vi "Archive files move dir.vi"(5 "hours old date mod(hours)":u8=255, 6 "error in":errorcluster, 7 "File path input cluster":T1={"Archive Location"=path "", "Archive Location 2"=path "<Not A Path>", "OutPut Path"=path "", "Directory(s) To Scan Files"=[]}, 8 "File Management":T2, 9 "Timing True to archive":bool) -> (0 "ErrorArray":errorcluster[][](array[cluster]), 1 "File path input cluster (out)":T1={"Archive Location"=path "", "Archive Location 2"=path "<Not A Path>", "OutPut Path"=path "", "Directory(s) To Scan Files"=[]})   [LabVIEW 2012]
uses:
  Controls/File Management.ctl
  Controls/File Path directories.ctl
  <vilib>/Utility/sysdir.llb/System Directory Type.ctl
panel:
  # "File Handling Method"
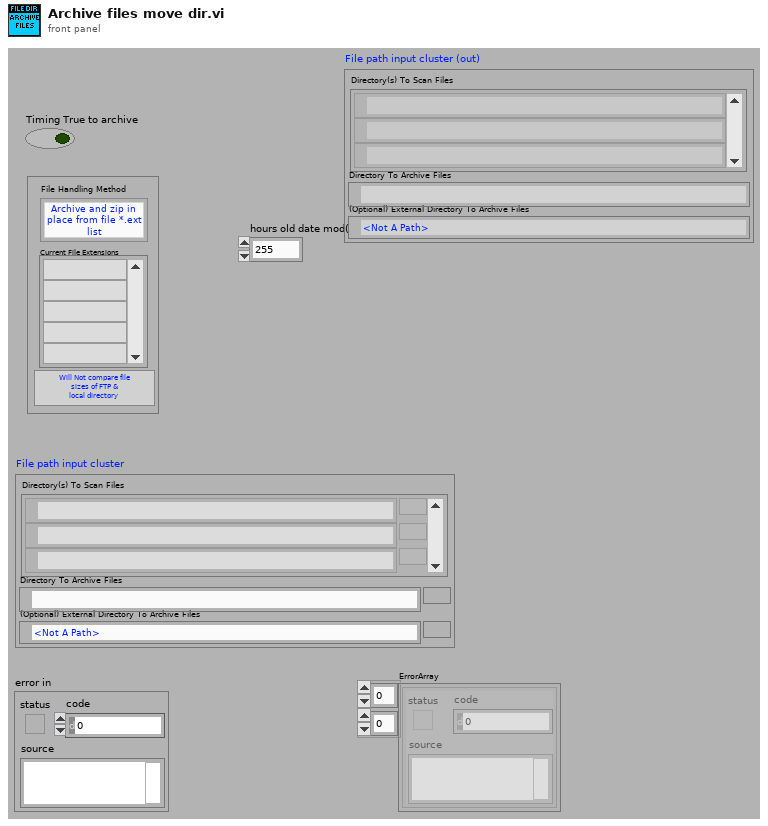
[diagram p1: front panel]
types:
  T1 = typedef "File Path directories.ctl" = cluster{"Archive Location":path, "Archive Location 2":path, "OutPut Path":path, "Directory(s) To Scan Files":path[]}
  T2 = typedef "File Management.ctl" = cluster{"Comp File Size":bool, "File Handle Method":enum16{"Archive and zip in place from file *.ext list", "Archive and zip ALL file Types to archive directory", "Archive and zip to archive directory from file *.ext list", "Perform no file management"}, "file extention list":string[]}
  T3 = enum16{"Archive and zip in place from file *.ext list", "Archive and zip ALL file Types to archive directory", "Archive and zip to archive directory from file *.ext list", "Perform no file management"}
  T4 = typedef "System Directory Type.ctl" = i32
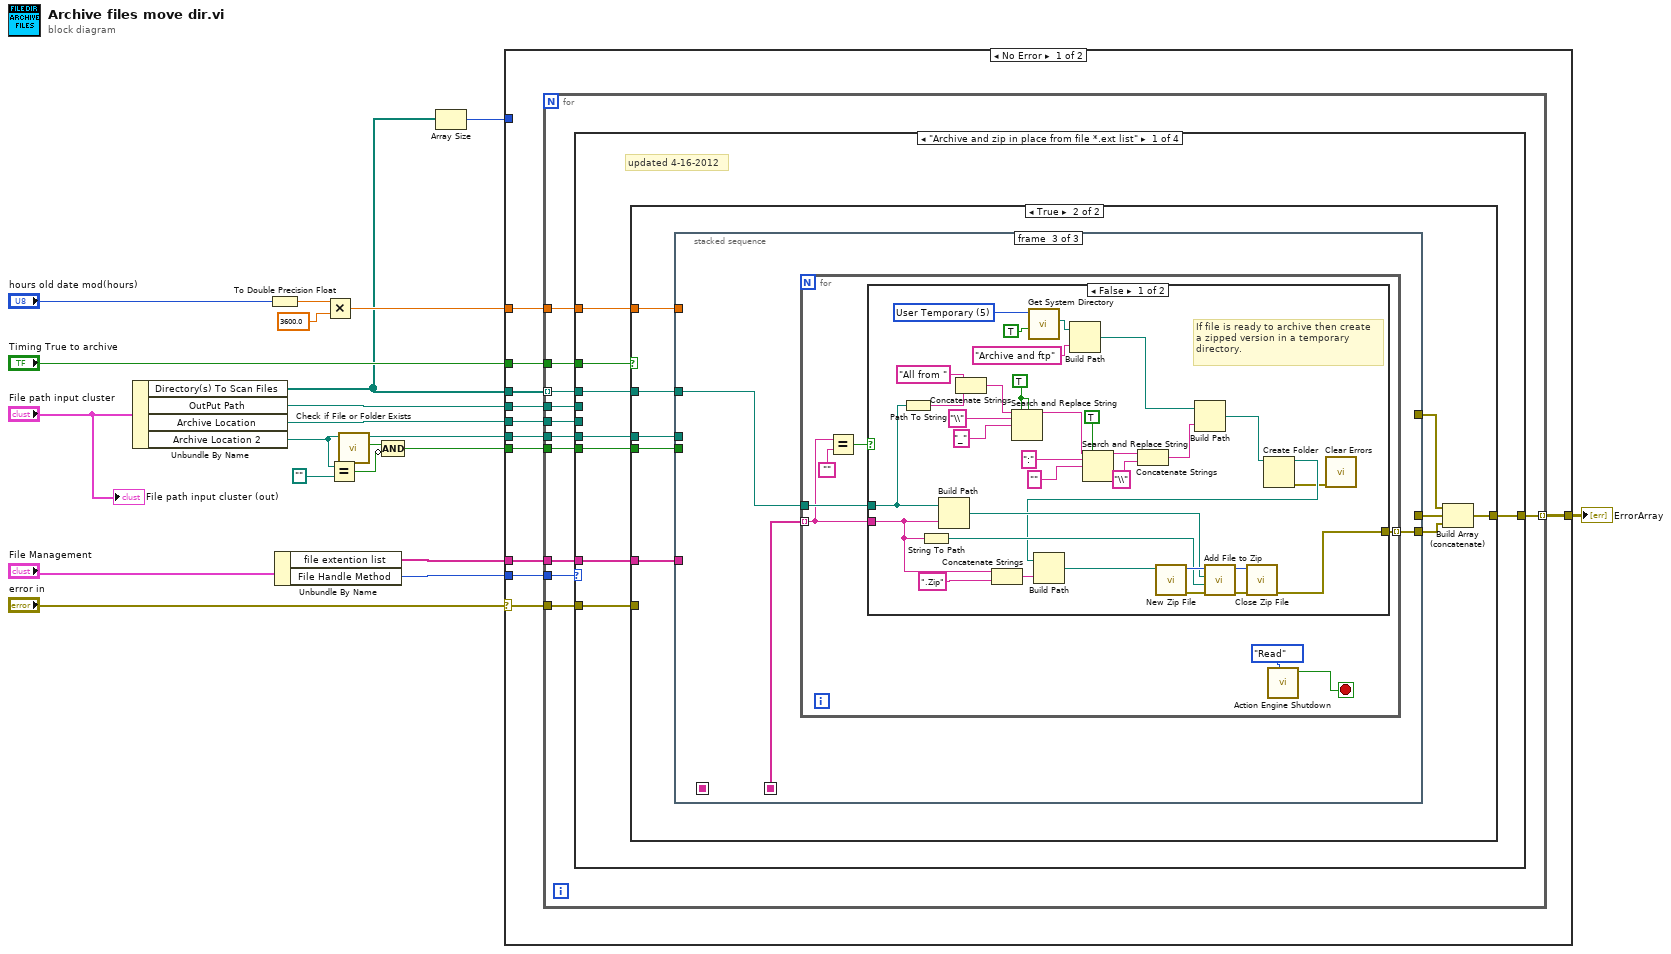
[diagram p0: block diagram]
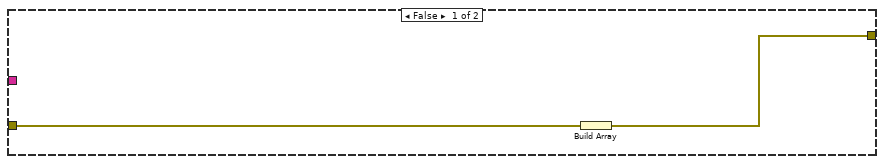
[diagram p2: hidden frame]
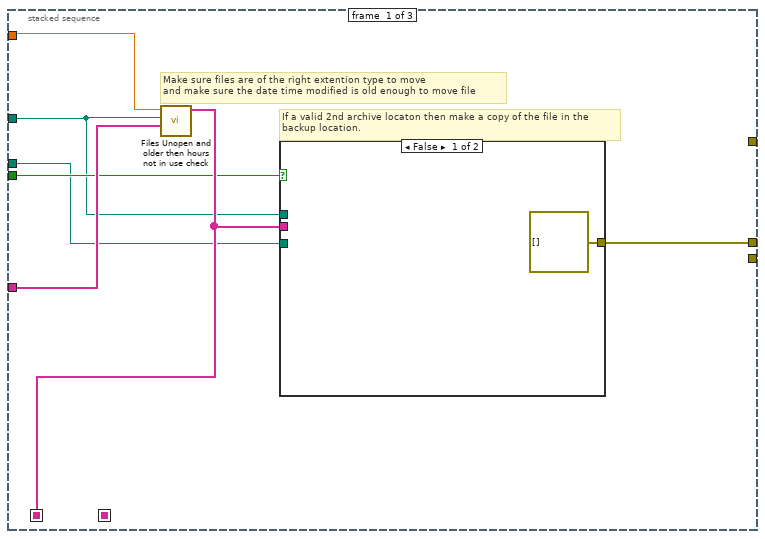
[diagram p3: hidden frame]
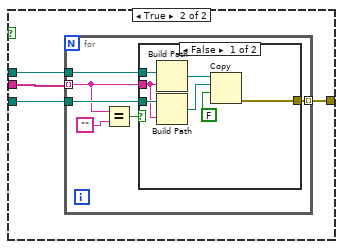
[diagram p4: hidden frame]
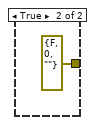
[diagram p5: hidden frame]
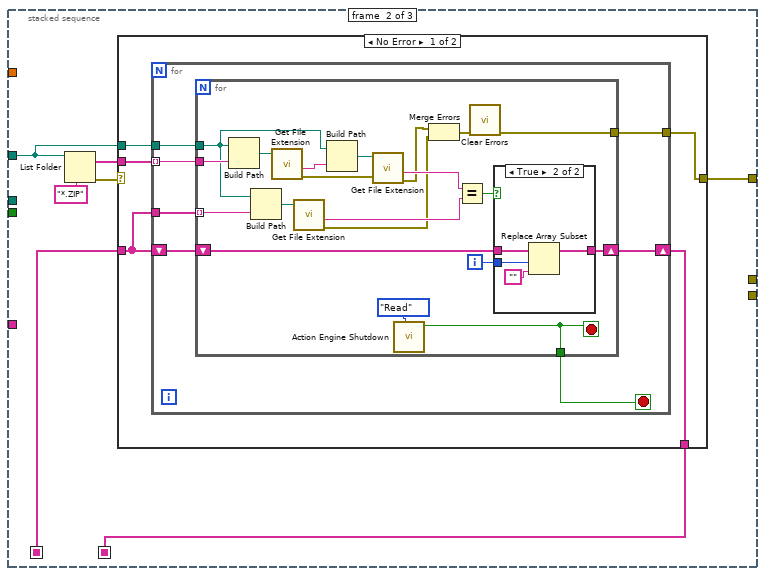
[diagram p6: hidden frame]
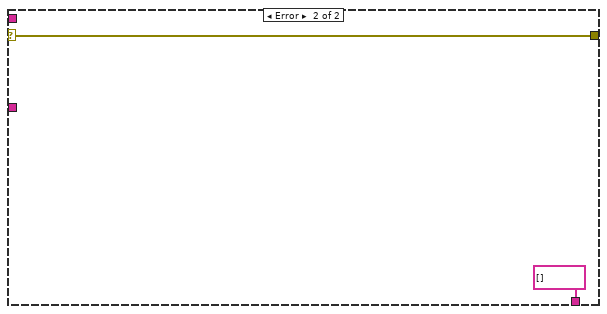
[diagram p8: hidden frame]
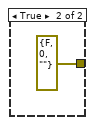
[diagram p9: hidden frame]
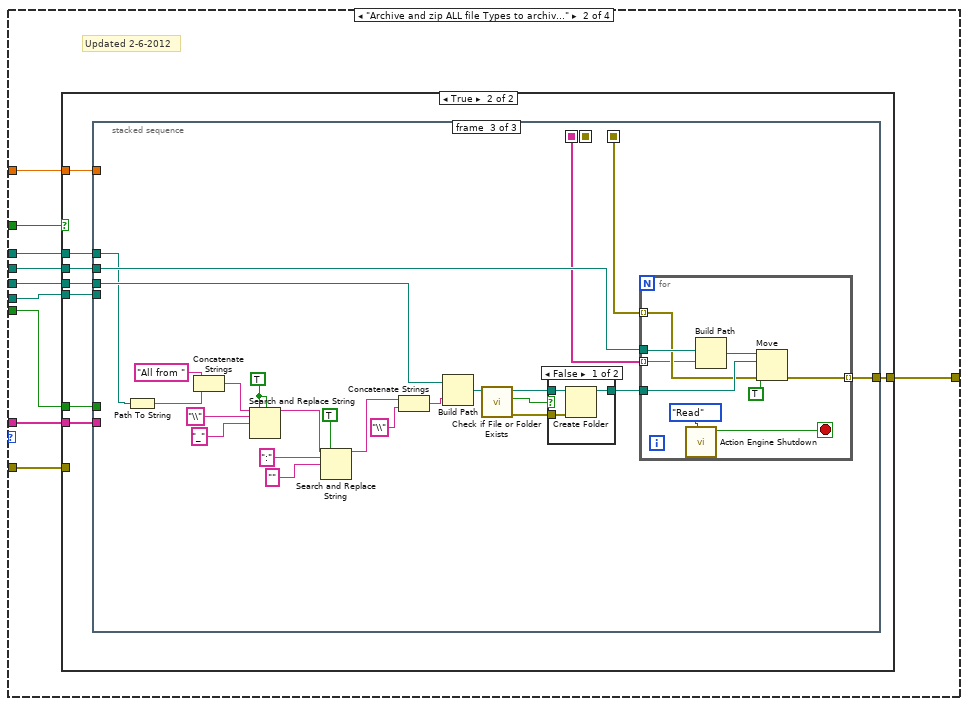
[diagram p10: hidden frame]
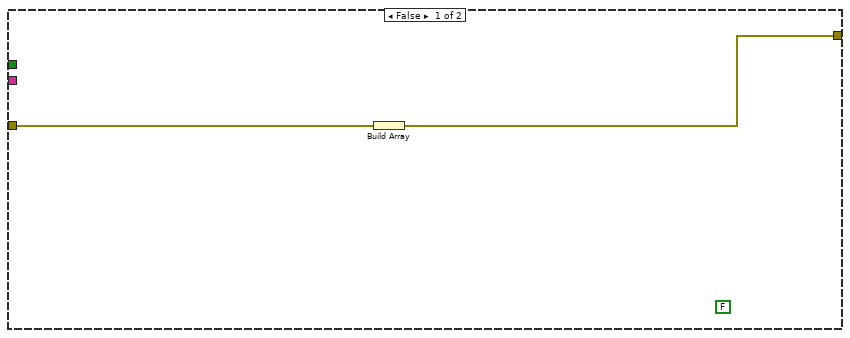
[diagram p11: hidden frame]
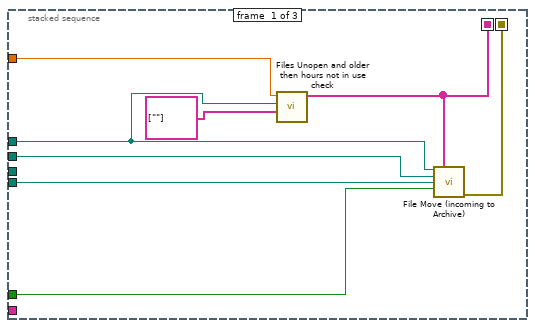
[diagram p12: hidden frame]
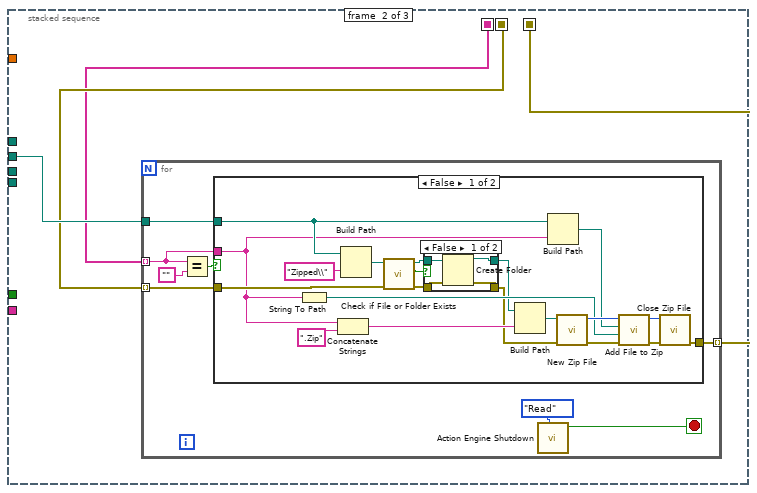
[diagram p13: hidden frame]
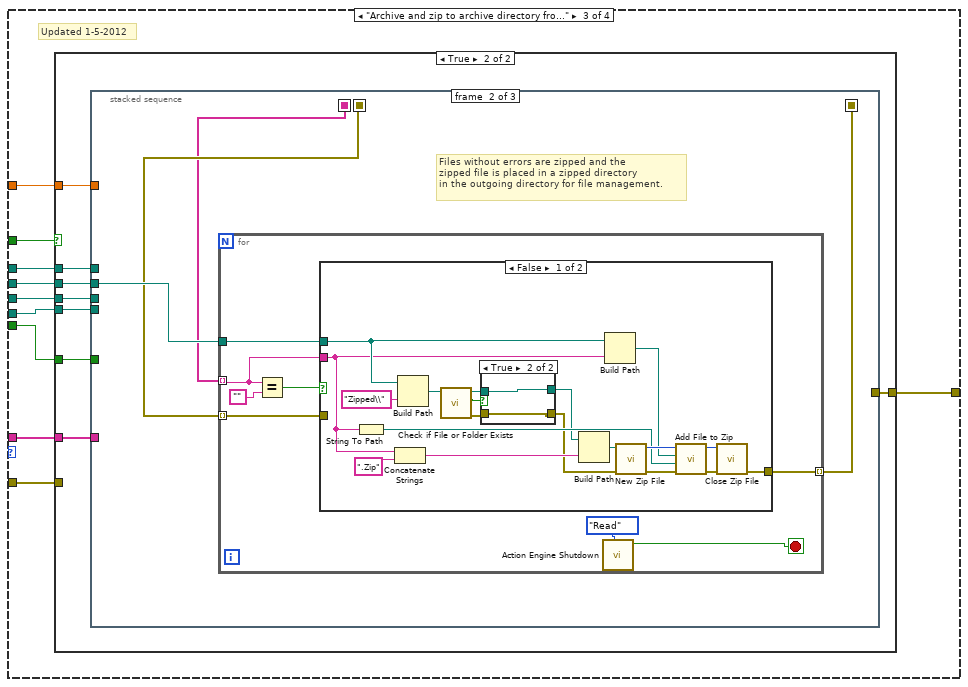
[diagram p17: hidden frame]
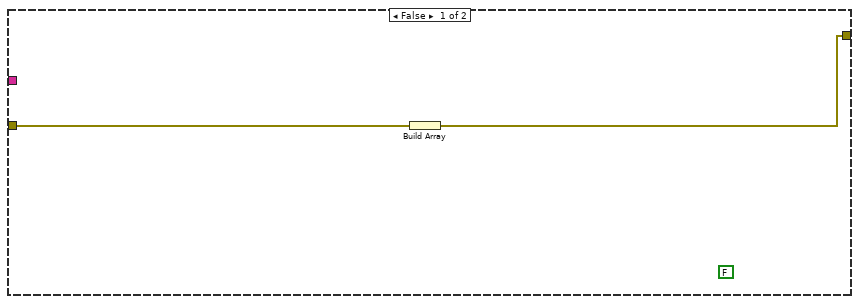
[diagram p18: hidden frame]
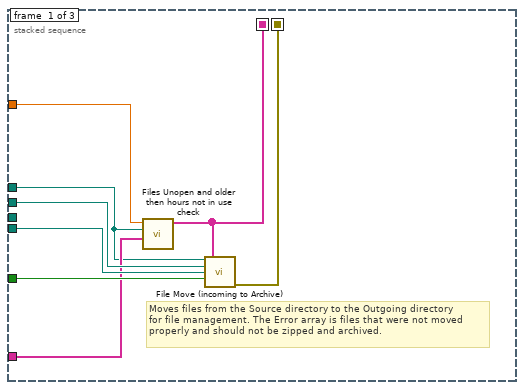
[diagram p19: hidden frame]
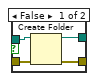
[diagram p20: hidden frame]
diagram:
  n1 = Unbundle By Name("File path input cluster") -> ("Directory(s) To Scan Files"=w3:path[], "OutPut Path"=w12:path, "Archive Location"=w11:path, "Archive Location 2"=w17:path)
  n2 = To Double Precision Float(number="hours old date mod(hours)") -> (double precision float=w6:dbl)
  n3 = Unbundle By Name("File Management") -> ("file extention list"=w18:string[], "File Handle Method"=w20:T3)
  n4 = Multiply(x=w6, y=3600.0) -> (x*y=w7:dbl)
  n5 = Equal?(x=w17, y=path "") -> (x = y?=w14:bool)
  n6 = call <vilib>:"Check if File or Folder Exists.vi"("path"=w17) -> ("file or folder exists?"=w15:bool, "dup path"=w10:path)  [unwired: 8 in, 1 out]
  n7 = Compound Arithmetic op=AND(w15, invert w14) -> (w9:bool)
  n8 = Array Size(array=w3) -> (size(s)=w2:i32)
  n9 = case shown="No Error" "error in" {
    selector: "error in" -> [w22 w381]
    tunnel: "Timing True to archive" -> [w32 _]
    tunnel: [w23 w379] -> w1
    tunnel: w20 -> [w31 _]
    tunnel: w18 -> [w30 _]
    tunnel: w3 -> [w29 _]
    tunnel: w12 -> [w28 _]
    tunnel: w11 -> [w27 _]
    tunnel: w10 -> [w26 _]
    tunnel: w9 -> [w25 _]
    tunnel: w7 -> [w24 _]
    tunnel: w2 -> [_ _]
    frame No Error {
      n10 = for {
        tunnel: w32 -> [w43]
        tunnel: w31 -> [w42]
        tunnel: w30 -> [w41]
        tunnel: w29 -> [w40] mode=indexing
        tunnel: w28 -> [w39]
        tunnel: w27 -> [w38]
        tunnel: w26 -> [w37]
        tunnel: w25 -> [w36]
        tunnel: w24 -> [w35]
        tunnel: [w34] -> w23 mode=indexing
        tunnel: w22 -> [w33]
        n11 = case shown="\"Archive and zip in place from file *.ext list\"" w42 {
          tunnel: w43 -> [w51 w188 w292 _]
          tunnel: w40 -> [w50 w187 w291 _]
          tunnel: w39 -> [_ w186 w290 _]
          tunnel: w38 -> [_ w185 w289 _]
          tunnel: w37 -> [w46 w184 w288 _]
          tunnel: w36 -> [w47 w183 w287 _]
          tunnel: w41 -> [w49 w182 w286 _]
          tunnel: w35 -> [w48 w181 w285 _]
          tunnel: [w44 w180 w284 w377] -> w34
          tunnel: w33 -> [w45 w179 w283 w378]
          frame "Archive and zip in place from file *.ext list" {
            # "updated 4-16-2012"
            n12 = case shown="True" w51 {
              tunnel: w50 -> [_ w62]
              tunnel: w49 -> [_ w61]
              tunnel: w48 -> [_ w60]
              tunnel: w47 -> [_ w59]
              tunnel: w46 -> [_ w58]
              tunnel: w45 -> [w53 _]
              tunnel: [w52 w54] -> w44
              frame False {
                n13 = Build Array(w53) -> (w52:errorcluster[])
              }
              frame True {
                n14 = stacked-sequence {
                  seq-local: [w67 _ _] -> [_ w93 _]
                  seq-local: [_ w90 _] -> [_ _ w136]
                  tunnel: w62 -> [w64 w91 w137]
                  tunnel: w61 -> [w68 _ _]
                  tunnel: w60 -> [w69 _ _]
                  tunnel: w59 -> [w66 _ _]
                  tunnel: w58 -> [w65 _ _]
                  tunnel: [w63 _ _] -> w57
                  tunnel: [_ w89 _] -> w56
                  tunnel: [_ _ w135] -> w55
                  frame #0 {
                    # "If a valid 2nd archive locaton then make a copy of the file in the \nbackup location."
                    # "Make sure files are of the right extention type to move\nand make sure the date time modified is old enough to move file"
                    n15 = call "Files Unopen and older then hours not in use check.vi"("file extention list"=w68, "Dir of Files to move and FTP"=w64, "Time (Hours) last mod must be older then"=w69) -> ("Files to Archive and FTP"=w67:string[])  [unwired: 8 in]
                    n16 = case shown="False" w66 {
                      tunnel: w67 -> [_ w74]
                      tunnel: w65 -> [_ w73]
                      tunnel: w64 -> [_ w72]
                      tunnel: [errorcluster[] [] w71] -> w63
                      frame False {
                      }
                      frame True {
                        n17 = for {
                          tunnel: w74 -> [w78] mode=indexing
                          tunnel: w72 -> [w80]
                          tunnel: w73 -> [w79]
                          tunnel: [w75] -> w71 mode=indexing
                          n18 = Equal?(x=w78, y="") -> (x = y?=w76:bool)
                          n19 = case shown="False" w76 {
                            tunnel: w80 -> [w87 _]
                            tunnel: w79 -> [w84 _]
                            tunnel: w78 -> [w82 _]
                            tunnel: [w81 errorcluster {"status"=FALSE, "code"=0, "source"=""} ("error out")] -> w75
                            frame False {
                              n20 = Build Path(base path=w87, name or relative path=w82) -> (appended path=w86:path)
                              n21 = Build Path(base path=w84, name or relative path=w82) -> (appended path=w83:path)
                              n22 = Copy(9:FALSE ("overwrite (F)"), 10:w83, 11:w86) -> (0:w81:errorcluster)  [unwired: 2 in, 2 out]
                            }
                            frame True {
                            }
                          }
                        }
                      }
                    }
                  }
                  frame #1 {
                    n23 = List Folder(path=w91, pattern="*.ZIP") -> (filenames=w94:string[], error out=w92:errorcluster)  [unwired: 2 in, 2 out]
                    n24 = case shown="No Error" w92 {
                      selector: w92 -> [_ w133]
                      tunnel: w94 -> [w100 _]
                      tunnel: w93 -> [w99 _]
                      tunnel: w91 -> [w98 _]
                      tunnel: [w97 string[] [] ("Files to Archive and FTP")] -> w90
                      tunnel: [w96 w133] -> w89
                      frame No Error {
                        n25 = for {
                          tunnel: w100 -> [w107] mode=indexing
                          tunnel: w99 -> [w106]
                          shift-right: [w104] -> w97
                          shift-left: w99 -> [w105]
                          tunnel: w98 -> [w103]
                          tunnel: [w101] -> w96
                          stop <- w102 stop-if-true
                          n26 = for {
                            tunnel: w106 -> [w119] mode=indexing
                            tunnel: w107 -> [w122]
                            shift-right: [w126] -> w104
                            shift-left: w105 -> [w124]
                            tunnel: w103 -> [w115]
                            tunnel: [w117] -> w102
                            tunnel: [w108] -> w101
                            i -> [w125]
                            stop <- w117 stop-if-true
                            n27 = Build Path(base path=w115, name or relative path=w122) -> (appended path=w123:path)
                            n28 = Build Path(base path=w115, name or relative path=w119) -> (appended path=w121:path)
                            n29 = call <vilib>:"Get File Extension.vi"("file"=w123) -> ("error out"=w113:errorcluster, "filename without extension"=w116:string)  [unwired: 7 in, 2 out]
                            n30 = call <vilib>:"Get File Extension.vi"("file"=w121) -> ("error out"=w111:errorcluster, "filename without extension"=w120:string)  [unwired: 7 in, 2 out]
                            n31 = Build Path(base path=w115, name or relative path=w116) -> (appended path=w114:path)
                            n32 = call <vilib>:"Get File Extension.vi"("error in (no error)"=w113, "file"=w114) -> ("error out"=w110:errorcluster, "filename without extension"=w112:string)  [unwired: 6 in, 2 out]
                            n33 = call "Action Engine Shutdown.vi"("Shutdown"=enum16{"Write", "Read"}."Read") -> ("Shutdown"=w117:bool)  [unwired: 9 in, 1 out]
                            n34 = Merge Errors(w110, w111) -> (w109:errorcluster)
                            n35 = Equal?(x=w112, y=w120) -> (x = y?=w127:bool)
                            n36 = call <vilib>:"Clear Errors.vi"("error in (no error)"=w109) -> ("error out"=w108:errorcluster)  [unwired: 6 in]
                            n37 = case shown="True" w127 {
                              tunnel: [w128 w132] -> w126
                              tunnel: w125 -> [_ w130]
                              tunnel: w124 -> [w128 w131]
                              frame False {
                              }
                              frame True {
                                n38 = Replace Array Subset(array=w131, new element="", index=w130) -> (w132:string[])
                              }
                            }
                          }
                        }
                      }
                      frame Error {
                      }
                    }
                  }
                  frame #2 {
                    n39 = for {
                      tunnel: w136 -> [w141] mode=indexing
                      tunnel: w137 -> [w144]
                      tunnel: [w138] -> w135 mode=indexing
                      stop <- w139 stop-if-true
                      n40 = Equal?(x=w141, y="") -> (x = y?=w143:bool)
                      n41 = case shown="False" w143 {
                        tunnel: w141 -> [w168 _]
                        tunnel: w144 -> [w152 _]
                        tunnel: [w145 errorcluster {"status"=FALSE, "code"=0, "source"=""} ("error IO")] -> w138
                        frame False {
                          w157 = TRUE ("replace all? (F)")
                          w164 = T4 5 items=["User Home"=0, "User Desktop"=1, "User Documents"=2, "User Application Data"=3, "User Preferences"=4, "User Temporary"=5, "Public Documents"=6, "Public Application Data"=7, "Public Preferences"=8, "Public Cache"=13, "System Core Libraries"=9, "System Installed Libraries"=10, "Application Files"=11, "Boot Volume Root"=12] ("system directory type")
                          # "If file is ready to archive then create\na zipped version in a temporary\ndirectory."
                          n42 = Path To String(path=w152) -> (string=w161:string)
                          n43 = String To Path(string=w168) -> (path=w173:path)
                          n44 = Build Path(base path=w152, name or relative path=w168) -> (appended path=w169:path)
                          n45 = Concatenate Strings("All from " ("name or relative path"), w161) -> (w160:string)
                          n46 = Concatenate Strings(w168, ".Zip" ("name or relative path")) -> (w170:string)
                          n47 = Search and Replace String(replace all?=w157, case sensitive?=w157, input string=w160, search string="\\" ("replace string (\"\")"), replace string="_" ("replace string (\"\")")) -> (result string=w154:string)  [unwired: 3 in, 3 out]
                          n48 = call <vilib>:"Get System Directory.vi"("create directory if not found? (F)"=TRUE, "system directory type"=w164) -> ("system directory"=w166:path)  [unwired: 9 in]
                          n49 = Build Path(base path=w166, name or relative path="Archive and ftp") -> (appended path=w151:path)
                          n50 = Search and Replace String(replace all?=TRUE ("replace all? (F)"), input string=w154, search string=":" ("replace string (\"\")"), replace string="" ("replace string (\"\")")) -> (result string=w150:string)  [unwired: 4 in, 3 out]
                          n51 = Concatenate Strings(w150, "\\" ("replace string (\"\")")) -> (w148:string)
                          n52 = Build Path(base path=w151, name or relative path=w148) -> (appended path=w147:path)
                          n53 = Create Folder(path (use dialog)=w147) -> (created path=w163:path, error out=w146:errorcluster)  [unwired: 2 in, 1 out]
                          n54 = Build Path(base path=w163, name or relative path=w170) -> (appended path=w172:path)
                          n55 = call <vilib>:"New Zip File.vi"("target"=w172) -> ("error out"=w174:errorcluster, "zip file out"=w177:i64)  [unwired: 4 in, 1 out]
                          n56 = call <vilib>:"Add File to Zip.vi"("error in (no error)"=w174, "destination path in zip"=w173, "source file path"=w169, "zip file in"=w177) -> ("error out"=w176:errorcluster, "zip file out"=w175:i64)  [unwired: 6 in]
                          n57 = call <vilib>:"Close Zip File.vi"("error in (no error)"=w176, "zip file in"=w175) -> ("error out"=w145:errorcluster)  [unwired: 5 in]
                          n58 = call <vilib>:"Clear Errors.vi"("error in (no error)"=w146) -> ()  [unwired: 6 in, 1 out]
                        }
                        frame True {
                        }
                      }
                      n59 = call "Action Engine Shutdown.vi"("Shutdown"=enum16{"Write", "Read"}."Read") -> ("Shutdown"=w139:bool)  [unwired: 9 in, 1 out]
                    }
                  }
                }
                n60 = Build Array (concatenate)(w56, w57, w55) -> (w54:errorcluster[])
              }
            }
          }
          frame "Archive and zip ALL file Types to archive directory" {
            # "Updated 2-6-2012"
            n61 = case shown="True" w188 {
              tunnel: w187 -> [_ w198]
              tunnel: w185 -> [_ w197]
              tunnel: w184 -> [_ w196]
              tunnel: w183 -> [_ w195]
              tunnel: w186 -> [_ w194]
              tunnel: w182 -> [_ w193]
              tunnel: w181 -> [_ w192]
              tunnel: [w189 w191] -> w180
              tunnel: w179 -> [w190 _]
              frame False {
                (unwired) FALSE ("Shutdown")
                n62 = Build Array(w190) -> (w189:errorcluster[])
              }
              frame True {
                n63 = stacked-sequence {
                  seq-local: [w199 _ _] -> [_ w207 w247]
                  seq-local: [w200 _ _] -> [_ w208 _]
                  seq-local: [_ w210 _] -> [_ _ w248]
                  tunnel: w198 -> [w202 _ w257]
                  tunnel: w197 -> [_ _ w266]
                  tunnel: w196 -> [w203 _ _]
                  tunnel: w195 -> [w204 _ _]
                  tunnel: w194 -> [w201 w209 w264]
                  tunnel: w193 -> [_ _ _]
                  tunnel: w192 -> [w205 _ _]
                  tunnel: [_ _ w246] -> w191
                  frame #0 {
                    n64 = call "Files Unopen and older then hours not in use check.vi"("file extention list"=string[] [""], "Dir of Files to move and FTP"=w202, "Time (Hours) last mod must be older then"=w205) -> ("Files to Archive and FTP"=w199:string[])  [unwired: 8 in]
                    n65 = call "File Move (incoming to Archive).vi"("source location of files"=w202, "Files to Archive and FTP IN"=w199, "outgoing directory"=w201, "redundant archive location"=w203, "Archive 2 valid path"=w204) -> ("Error OUT array"=w200:errorcluster[])  [unwired: 10 in]
                  }
                  frame #1 {
                    n66 = for {
                      tunnel: w209 -> [w217]
                      tunnel: [w218] -> w210 mode=indexing
                      tunnel: w208 -> [w216] mode=indexing
                      tunnel: w207 -> [w211] mode=indexing
                      stop <- w212 stop-if-true
                      n67 = Equal?(x=w211, y="") -> (x = y?=w215:bool)
                      n68 = case shown="False" w215 {
                        tunnel: [w233 w245] -> w218
                        tunnel: w217 -> [w228 _]
                        tunnel: w216 -> [w220 w245]
                        tunnel: w211 -> [w219 _]
                        frame False {
                          n69 = String To Path(string=w219) -> (path=w234:path)
                          n70 = Concatenate Strings(w219, ".Zip" ("name or relative path")) -> (w230:string)
                          n71 = Build Path(base path=w228, name or relative path="Zipped\\") -> (appended path=w226:path)
                          n72 = call <vilib>:"Check if File or Folder Exists.vi"("error in (no error)"=w220, "path"=w226) -> ("error out"=w222:errorcluster, "file or folder exists?"=w225:bool, "dup path"=w224:path)  [unwired: 7 in]
                          n73 = case shown="False" w225 {
                            tunnel: w224 -> [w242 w244]
                            tunnel: [w241 w244] -> w223
                            tunnel: w222 -> [w240 w243]
                            tunnel: [w239 w243] -> w221
                            frame False {
                              n74 = Create Folder(path (use dialog)=w242, error in=w240) -> (created path=w241:path, error out=w239:errorcluster)  [unwired: 1 in, 1 out]
                            }
                            frame True {
                            }
                          }
                          n75 = Build Path(base path=w223, name or relative path=w230) -> (appended path=w232:path)
                          n76 = Build Path(base path=w228, name or relative path=w219) -> (appended path=w229:path)
                          n77 = call <vilib>:"New Zip File.vi"("error in (no error)"=w221, "target"=w232) -> ("error out"=w235:errorcluster, "zip file out"=w238:i64)  [unwired: 3 in, 1 out]
                          n78 = call <vilib>:"Add File to Zip.vi"("error in (no error)"=w235, "destination path in zip"=w234, "source file path"=w229, "zip file in"=w238) -> ("error out"=w237:errorcluster, "zip file out"=w236:i64)  [unwired: 6 in]
                          n79 = call <vilib>:"Close Zip File.vi"("error in (no error)"=w237, "zip file in"=w236) -> ("error out"=w233:errorcluster)  [unwired: 5 in]
                        }
                        frame True {
                        }
                      }
                      n80 = call "Action Engine Shutdown.vi"("Shutdown"=enum16{"Write", "Read"}."Read") -> ("Shutdown"=w212:bool)  [unwired: 9 in, 1 out]
                    }
                  }
                  frame #2 {
                    w255 = TRUE ("replace all? (F)")
                    n81 = Path To String(path=w257) -> (string=w262:string)
                    n82 = Concatenate Strings("All from " ("name or relative path"), w262) -> (w261:string)
                    n83 = Search and Replace String(replace all?=w255, case sensitive?=w255, input string=w261, search string="\\" ("replace string (\"\")"), replace string="_" ("replace string (\"\")")) -> (result string=w251:string)  [unwired: 3 in, 3 out]
                    n84 = Search and Replace String(replace all?=TRUE ("replace all? (F)"), input string=w251, search string=":" ("replace string (\"\")"), replace string="" ("replace string (\"\")")) -> (result string=w250:string)  [unwired: 4 in, 3 out]
                    n85 = Concatenate Strings(w250, "\\" ("replace string (\"\")")) -> (w254:string)
                    n86 = Build Path(base path=w266, name or relative path=w254) -> (appended path=w269:path)
                    n87 = call <vilib>:"Check if File or Folder Exists.vi"("path"=w269) -> ("error out"=w258:errorcluster, "file or folder exists?"=w268:bool, "dup path"=w267:path)  [unwired: 8 in]
                    n88 = case shown="False" w268 {
                      tunnel: w267 -> [w281 w282]
                      tunnel: [w280 w282] -> w265
                      tunnel: w258 -> [w279 _]
                      frame False {
                        n89 = Create Folder(path (use dialog)=w281, error in=w279) -> (created path=w280:path)  [unwired: 1 in, 2 out]
                      }
                      frame True {
                      }
                    }
                    n90 = for {
                      tunnel: w265 -> [w278]
                      tunnel: w264 -> [w275]
                      tunnel: w248 -> [w274] mode=indexing
                      tunnel: w247 -> [w271] mode=indexing
                      tunnel: [w270] -> w246 mode=indexing
                      stop <- w272 stop-if-true
                      n91 = call "Action Engine Shutdown.vi"("Shutdown"=enum16{"Write", "Read"}."Read") -> ("Shutdown"=w272:bool)  [unwired: 9 in, 1 out]
                      n92 = Build Path(base path=w275, name or relative path=w271) -> (appended path=w277:path)
                      n93 = Move(source path=w277, error in=w274, 9:TRUE ("overwrite (F)"), 10:w278) -> (error out=w270:errorcluster)  [unwired: 1 in, 2 out]
                    }
                  }
                }
              }
            }
          }
          frame "Archive and zip to archive directory from file *.ext list" {
            # "Updated 1-5-2012"
            n94 = case shown="True" w292 {
              tunnel: w291 -> [_ w302]
              tunnel: w289 -> [_ w301]
              tunnel: w288 -> [_ w300]
              tunnel: w287 -> [_ w299]
              tunnel: w290 -> [_ w298]
              tunnel: w286 -> [_ w297]
              tunnel: w285 -> [_ w296]
              tunnel: [w293 w295] -> w284
              tunnel: w283 -> [w294 _]
              frame False {
                (unwired) FALSE ("Shutdown")
                n95 = Build Array(w294) -> (w293:errorcluster[])
              }
              frame True {
                n96 = stacked-sequence {
                  seq-local: [w303 _ _] -> [_ w311 w350]
                  seq-local: [w306 _ _] -> [_ w313 _]
                  seq-local: [_ w312 _] -> [_ _ w351]
                  tunnel: w302 -> [w304 _ _]
                  tunnel: w301 -> [_ _ w353]
                  tunnel: w300 -> [w309 _ _]
                  tunnel: w299 -> [w310 _ _]
                  tunnel: w298 -> [w308 w314 w352]
                  tunnel: w297 -> [w305 _ _]
                  tunnel: w296 -> [w307 _ _]
                  tunnel: [_ _ w349] -> w295
                  frame #0 {
                    # "Moves files from the Source directory to the Outgoing directory\nfor file management. The Error array is files that were not moved\nproperly and should not be zipped and archived."
                    n97 = call "Files Unopen and older then hours not in use check.vi"("file extention list"=w305, "Dir of Files to move and FTP"=w304, "Time (Hours) last mod must be older then"=w307) -> ("Files to Archive and FTP"=w303:string[])  [unwired: 8 in]
                    n98 = call "File Move (incoming to Archive).vi"("source location of files"=w304, "Files to Archive and FTP IN"=w303, "outgoing directory"=w308, "redundant archive location"=w309, "Archive 2 valid path"=w310) -> ("Error OUT array"=w306:errorcluster[])  [unwired: 10 in]
                  }
                  frame #1 {
                    # "Files without errors are zipped and the \nzipped file is placed in a zipped directory\nin the outgoing directory for file management."
                    n99 = for {
                      tunnel: w314 -> [w322]
                      tunnel: w313 -> [w318] mode=indexing
                      tunnel: [w319] -> w312 mode=indexing
                      tunnel: w311 -> [w315] mode=indexing
                      stop <- w316 stop-if-true
                      n100 = Equal?(x=w315, y="") -> (x = y?=w321:bool)
                      n101 = case shown="False" w321 {
                        tunnel: w322 -> [w332 _]
                        tunnel: [w324 errorcluster {"status"=TRUE, "code"=0, "source"=""} ("error out")] -> w319
                        tunnel: w318 -> [_ _]
                        tunnel: w315 -> [w323 _]
                        frame False {
                          n102 = String To Path(string=w323) -> (path=w337:path)
                          n103 = Concatenate Strings(w323, ".Zip" ("name or relative path")) -> (w334:string)
                          n104 = Build Path(base path=w332, name or relative path="Zipped\\") -> (appended path=w330:path)
                          n105 = call <vilib>:"Check if File or Folder Exists.vi"("path"=w330) -> ("error out"=w326:errorcluster, "file or folder exists?"=w329:bool, "dup path"=w328:path)  [unwired: 8 in]
                          n106 = case shown="True" w329 {
                            tunnel: w328 -> [w345 w347]
                            tunnel: [w344 w347] -> w327
                            tunnel: w326 -> [w343 w346]
                            tunnel: [w342 w346] -> w325
                            frame False {
                              n107 = Create Folder(path (use dialog)=w345, error in=w343) -> (created path=w344:path, error out=w342:errorcluster)  [unwired: 1 in, 1 out]
                            }
                            frame True {
                            }
                          }
                          n108 = Build Path(base path=w327, name or relative path=w334) -> (appended path=w336:path)
                          n109 = Build Path(base path=w332, name or relative path=w323) -> (appended path=w333:path)
                          n110 = call <vilib>:"New Zip File.vi"("error in (no error)"=w325, "target"=w336) -> ("error out"=w338:errorcluster, "zip file out"=w341:i64)  [unwired: 3 in, 1 out]
                          n111 = call <vilib>:"Add File to Zip.vi"("error in (no error)"=w338, "destination path in zip"=w337, "source file path"=w333, "zip file in"=w341) -> ("error out"=w340:errorcluster, "zip file out"=w339:i64)  [unwired: 6 in]
                          n112 = call <vilib>:"Close Zip File.vi"("error in (no error)"=w340, "zip file in"=w339) -> ("error out"=w324:errorcluster)  [unwired: 5 in]
                        }
                        frame True {
                        }
                      }
                      n113 = call "Action Engine Shutdown.vi"("Shutdown"=enum16{"Write", "Read"}."Read") -> ("Shutdown"=w316:bool)  [unwired: 9 in, 1 out]
                    }
                  }
                  frame #2 {
                    # "this Error array \nis the result of \nfiles that failed\nat zipping."
                    n114 = for {
                      tunnel: w353 -> [w360]
                      tunnel: w352 -> [w359]
                      tunnel: w351 -> [w358] mode=indexing
                      tunnel: w350 -> [w357] mode=indexing
                      tunnel: [w354] -> w349 mode=indexing
                      stop <- w355 stop-if-true
                      n115 = case shown="No Error" w358 {
                        selector: w358 -> [_ w376]
                        tunnel: w360 -> [w372 _]
                        tunnel: w359 -> [w366 _]
                        tunnel: w357 -> [w365 _]
                        tunnel: [w361 w376] -> w354
                        frame No Error {
                          n116 = Build Path(base path=w366, name or relative path=w365) -> (appended path=w364:path)
                          n117 = call <vilib>:"Get File Extension.vi"("file"=w364) -> ("lowercase file extension"=w363:string)  [unwired: 7 in, 3 out]
                          n118 = To Upper Case(1:w363) -> (0:w362:string)
                          n119 = Build Path(base path=w372, name or relative path=w362) -> (appended path=w371:path)
                          n120 = call <vilib>:"Check if File or Folder Exists.vi"("path"=w371) -> ("file or folder exists?"=w370:bool, "dup path"=w369:path)  [unwired: 8 in, 1 out]
                          n121 = case shown="False" w370 {
                            tunnel: w369 -> [w374 w375]
                            tunnel: [w373 w375] -> w368
                            frame False {
                              n122 = Create Folder(path (use dialog)=w374) -> (created path=w373:path)  [unwired: 2 in, 2 out]
                            }
                            frame True {
                            }
                          }
                          n123 = Move(source path=w364, 9:TRUE ("overwrite (F)"), 10:w368) -> (error out=w361:errorcluster)  [unwired: 2 in, 2 out]
                        }
                        frame Error {
                        }
                      }
                      n124 = call "Action Engine Shutdown.vi"("Shutdown"=enum16{"Write", "Read"}."Read") -> ("Shutdown"=w355:bool)  [unwired: 9 in, 1 out]
                    }
                  }
                }
              }
            }
          }
          frame "Perform no file management", Default {
            n125 = Build Array(w378) -> (w377:errorcluster[])
          }
        }
      }
    }
    frame Error {
      n126 = Build Array(w381) -> (w380:errorcluster[])
      n127 = Build Array(w380) -> (w379:errorcluster[][])
    }
  }
  "ErrorArray" <- w1
  "File path input cluster (out)" <- "File path input cluster"
